vi "Config-Display-List.vi"(8 "error in (no error)":errorcluster, 9 "data variables":cluster{"variable1":string, "variable2":string}, 10 "list (max 8 elements)":string[](array[string]), 11 "VISA session":refnum<visa-resource-name>) -> (0 "error out":errorcluster)   [LabVIEW 2016, in "Agilent 415X Series.lvlib"]
doc: "This VI configures the instrument for LIST display mode. Executing this VI will automatically place the instrument in LIST display mode."
uses:
  Agilent 415X Series.lvlib
panel:
  # "This VI selects LIST display mode automatically."
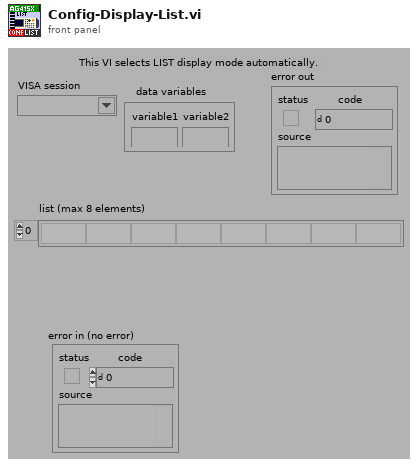
[diagram p1: front panel]
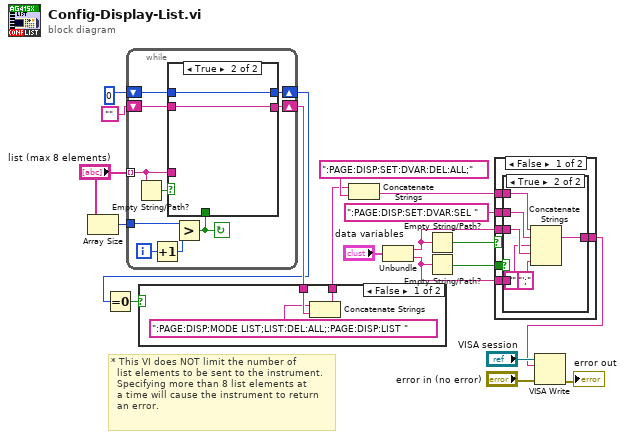
[diagram p0: block diagram]
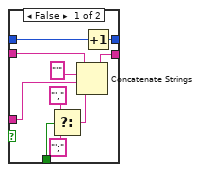
[diagram p2: hidden frame]
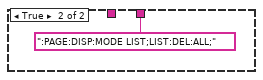
[diagram p3: hidden frame]
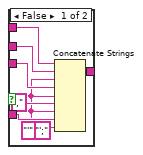
[diagram p4: hidden frame]
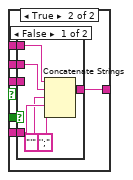
[diagram p5: hidden frame]
diagram:
  # "* This VI does NOT limit the number of\n  list elements to be sent to the instrument.\n  Specifying more than 8 list elements at\n  a time will cause the instrument to return\n  an error."
  n1 = Array Size(array="list (max 8 elements)") -> (size(s)=w2:i32)
  n2 = while {
    shift-left: 0 -> [w22]
    shift-right: [w21] -> w1
    shift-left: "" -> [w24]
    shift-right: [w23] -> w8
    tunnel: w2 -> [w29]
    tunnel: "list (max 8 elements)" -> [w25] mode=indexing
    i -> [w30]
    stop <- w27 continue-if-true
    n3 = Empty String/Path?(string/path=w25) -> (empty?=w26:bool)
    n4 = Increment(x=w30) -> (x+1=w28:i32)
    n5 = Greater?(x=w29, y=w28) -> (0:w27:bool)
    n6 = case shown="True" w26 {
      tunnel: w27 -> [w36 _]
      tunnel: w25 -> [w35 _]
      tunnel: w24 -> [w34 w42]
      tunnel: [w33 w42] -> w23
      tunnel: [w31 w41] -> w21
      tunnel: w22 -> [w32 w41]
      frame False {
        n7 = Select(t="',", s=w36, f="';") -> (s? t:f=w40:string)
        n8 = Concatenate Strings(w34, "'", w35, w40) -> (w33:string)
        n9 = Increment(x=w32) -> (x+1=w31:i32)
      }
      frame True {
      }
    }
  }
  n10 = Equal To 0?(x=w1) -> (x = 0?=w9:bool)
  n11 = case shown="False" w9 {
    tunnel: w8 -> [w45 _]
    tunnel: [w43 ":PAGE:DISP:MODE LIST;LIST:DEL:ALL;"] -> w7
    frame False {
      n12 = Concatenate Strings(":PAGE:DISP:MODE LIST;LIST:DEL:ALL;:PAGE:DISP:LIST ", w45) -> (w43:string)
    }
    frame True {
    }
  }
  n13 = Concatenate Strings(w7, ":PAGE:DISP:SET:DVAR:DEL:ALL;") -> (w14:string)
  n14 = Unbundle("data variables") -> ("variable1"=w17:string, "variable2"=w16:string)
  n15 = Empty String/Path?(string/path=w17) -> (empty?=w19:bool)
  n16 = Empty String/Path?(string/path=w16) -> (empty?=w18:bool)
  n17 = case shown="False" w19 {
    tunnel: w18 -> [w52 w72]
    tunnel: w17 -> [w51 w71]
    tunnel: w16 -> [w50 w70]
    tunnel: w14 -> [w49 w69]
    tunnel: ":PAGE:DISP:SET:DVAR:SEL " -> [w48 w68]
    tunnel: [w47 w67] -> w6
    frame False {
      n18 = case shown="True" w52 {
        tunnel: w51 -> [w57 w63]
        tunnel: w50 -> [w54 _]
        tunnel: w49 -> [w60 w66]
        tunnel: w48 -> [w59 w65]
        tunnel: [w58 w64] -> w47
        frame False {
          w53 = "'"
          n19 = Concatenate Strings(w60, w59, w53, w57, w53, ",", w53, w54, "';") -> (w58:string)
        }
        frame True {
          n20 = Concatenate Strings(w66, w65, "'", w63, "';") -> (w64:string)
        }
      }
    }
    frame True {
      n21 = case shown="False" w72 {
        tunnel: w71 -> [_ _]
        tunnel: w70 -> [w75 _]
        tunnel: w69 -> [w78 w79]
        tunnel: w68 -> [w77 _]
        tunnel: [w76 w79] -> w67
        frame False {
          n22 = Concatenate Strings(w78, w77, "'", w75, "';") -> (w76:string)
        }
        frame True {
        }
      }
    }
  }
  n23 = VISA Write(VISA resource name="VISA session", write buffer=w6, error in (no error)="error in (no error)") -> (error out=→"error out":errorcluster)  [unwired: 2 out]
